vi "unflatten PID.vi"(10 "Identifier":string, 11 "Data to Unwrap":string) -> (3 "PID Loops":T1={"ID"="", "Setpoint"=refnum, "Process Variable"=refnum, "Output"=refnum, "PID gains"={"proportional gain (Kc)"=1.0, "integral time (Ti, min)"=0.01, "derivative time (Td, min)"=0.0}, "output range"={"output high"=100.0, "output low"=-100.0}} {"output range"."output low" format="%.2f"; "output range"."output high" format="%.2f"})   [LabVIEW 2014, in "Tagbus PID Module configuration.lvclass"]
uses:
  Tagbus PID Module configuration.lvclass
  <vilib>/NI/Tag Bus Module Framework/channel/TBM channel.lvclass
  <vilib>/NI/Configuration Framework/serializable configuration/NISE_CEF_serializable configuration.lvclass
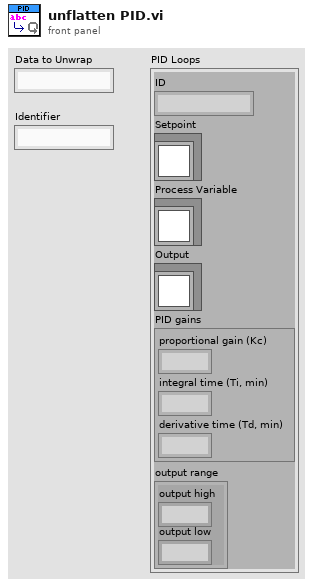
[diagram p1: front panel]
types:
  T1 = cluster{"ID":string, "Setpoint":refnum<class "TBM channel.lvclass">, "Process Variable":refnum<class "TBM channel.lvclass">, "Output":refnum<class "TBM channel.lvclass">, "PID gains":cluster{"proportional gain (Kc)":dbl, "integral time (Ti, min)":dbl, "derivative time (Td, min)":dbl}, "output range":cluster{"output high":dbl, "output low":dbl}}
  T2 = enum16{"Setpoint", "Process Variable", "Output", "Gains", "Range"}
  T3 = cluster{"proportional gain (Kc)":dbl, "integral time (Ti, min)":dbl, "derivative time (Td, min)":dbl}
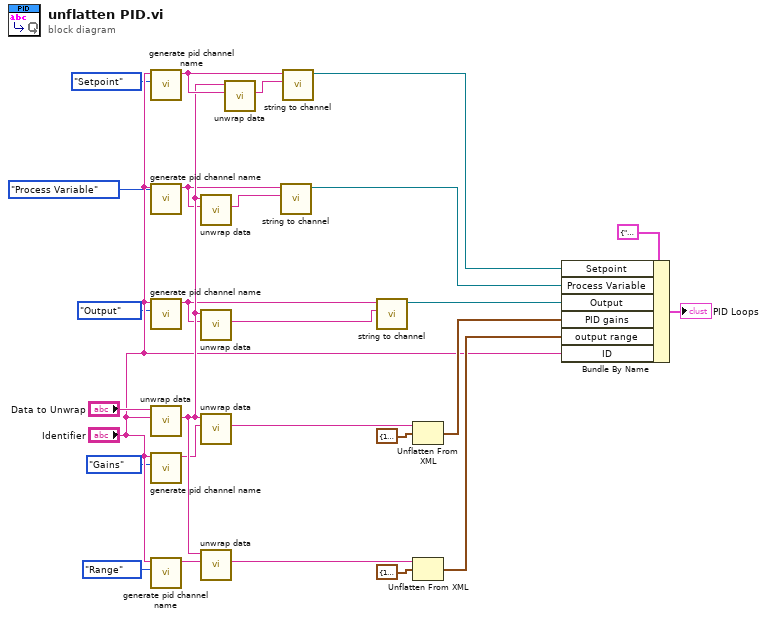
[diagram p0: block diagram]
diagram:
  n1 = call "generate pid channel name.vi"("Property"=T2."Setpoint", "Identifier"="Identifier") -> ("Property Name"=w18:string)  [unwired: 9 in]
  n2 = call "generate pid channel name.vi"("Property"=T2."Process Variable", "Identifier"="Identifier") -> ("Property Name"=w10:string)  [unwired: 9 in]
  n3 = call "generate pid channel name.vi"("Property"=T2."Output", "Identifier"="Identifier") -> ("Property Name"=w9:string)  [unwired: 9 in]
  n4 = call <vilib>:"unwrap data.vi"("identifier"="Identifier", "data to unwrap"="Data to Unwrap") -> ("unwrapped data"=w17:string)  [unwired: 8 in, 1 out]
  n5 = call "generate pid channel name.vi"("Property"=T2."Gains", "Identifier"="Identifier") -> ("Property Name"=w8:string)  [unwired: 9 in]
  n6 = call "generate pid channel name.vi"("Property"=T2."Range", "Identifier"="Identifier") -> ("Property Name"=w7:string)  [unwired: 9 in]
  n7 = call <vilib>:"unwrap data.vi"("identifier"=w10, "data to unwrap"=w17) -> ("unwrapped data"=w20:string)  [unwired: 8 in, 1 out]
  n8 = call <vilib>:"unwrap data.vi"("identifier"=w9, "data to unwrap"=w17) -> ("unwrapped data"=w21:string)  [unwired: 8 in, 1 out]
  n9 = call <vilib>:"unwrap data.vi"("identifier"=w8, "data to unwrap"=w17) -> ("unwrapped data"=w15:string)  [unwired: 8 in, 1 out]
  n10 = call <vilib>:"unwrap data.vi"("identifier"=w7, "data to unwrap"=w17) -> ("unwrapped data"=w12:string)  [unwired: 8 in, 1 out]
  n11 = call <vilib>:"unwrap data.vi"("identifier"=w18, "data to unwrap"=w17) -> ("unwrapped data"=w19:string)  [unwired: 8 in, 1 out]
  n12 = call <vilib>:"string to channel.vi"("channel data"=w20, "identifier"=w10) -> ("channel in"=w24:refnum<class "TBM channel.lvclass">)  [unwired: 9 in]
  n13 = call <vilib>:"string to channel.vi"("channel data"=w19, "identifier"=w18) -> ("channel in"=w23:refnum<class "TBM channel.lvclass">)  [unwired: 9 in]
  n14 = call <vilib>:"string to channel.vi"("channel data"=w21, "identifier"=w9) -> ("channel in"=w25:refnum<class "TBM channel.lvclass">)  [unwired: 9 in]
  n15 = Unflatten From XML(xml string=w15, type=T3 {"proportional gain (Kc)"=1.0, "integral time (Ti, min)"=0.01, "derivative time (Td, min)"=0.0} ("PID gains")) -> (value=w27:T3)  [unwired: 1 in, 1 out]
  n16 = Unflatten From XML(xml string=w12, type=cluster{"output high":dbl, "output low":dbl} {"output high"=100.0, "output low"=-100.0} ("output range")) -> (value=w13:cluster{"output high":dbl, "output low":dbl})  [unwired: 1 in, 1 out]
  n17 = Bundle By Name(cluster=T1 {"ID"="", "Setpoint"=refnum, "Process Variable"=refnum, "Output"=refnum, "PID gains"={"proportional gain (Kc)"=1.0, "integral time (Ti, min)"=0.01, "derivative time (Td, min)"=0.0}, "output range"={"output high"=100.0, "output low"=-100.0}} ("Channels"), "Setpoint"=w23, "Process Variable"=w24, "Output"=w25, "PID gains"=w27, "output range"=w13, "ID"="Identifier") -> (→"PID Loops":T1)
